vi "Camera Parameter to 3D Projection Matrix.vi"(0 "Size":T2, 1 "Far (Default: 100)":dbl=100.0 format="%#_13g", 3 "Camera Matrix":T1, 4 "Near (Default: 0.01)":dbl=0.01 format="%#_13g") -> (2 "Bounds":T3, 5 "3D-Control Projection Matrix":sgl[][](array[numeric]))   [LabVIEW 2020, in "g_ar_toolkit.ar.lvlib"]
uses:
  g_ar_toolkit.ar.lvlib
  <vilib>/Utility/miscctls.llb/LVBoundsTypeDef.ctl
  g_ar_toolkit.common/Image Size (Integer).ctl
  g_ar_toolkit.common/Camera Matrix.ctl
  g_ar_toolkit.common/g_ar_toolkit.common.lvlib
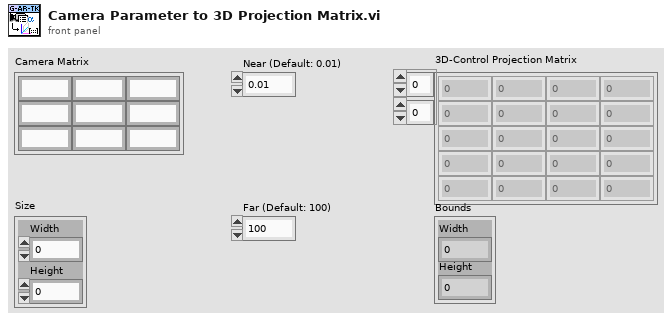
[diagram p1: front panel]
types:
  T1 = typedef "g_ar_toolkit.common.lvlib/Camera Matrix.ctl" = cluster{"m 0,0":dbl, "m 0,1":dbl, "m 0,2":dbl, "m 1,0":dbl, "m 1,1":dbl, "m 1,2":dbl, "m 2,0":dbl, "m 2,1":dbl, "m 2,2":dbl}
  T2 = typedef "g_ar_toolkit.common.lvlib/Image Size (Integer).ctl" = cluster{"Width":u16, "Height":u16}
  T3 = typedef "LVBoundsTypeDef.ctl" = cluster{"Width":u32, "Height":u32}
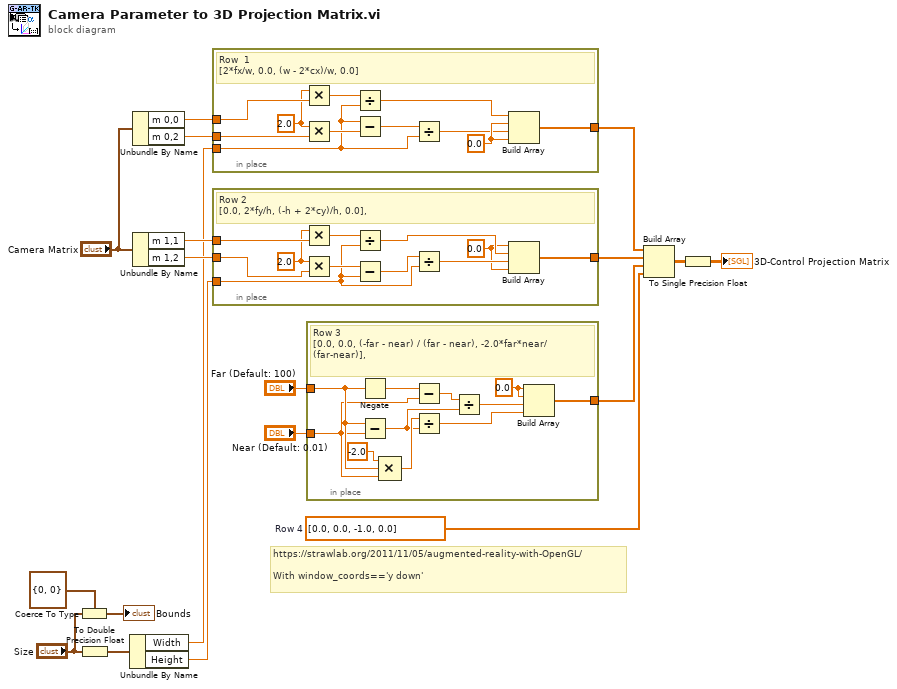
[diagram p0: block diagram]
diagram:
  w17 = dbl[] [0.0, 0.0, -1.0, 0.0]  # Row 4
  # "https://strawlab.org/2011/11/05/augmented-reality-with-OpenGL/\n\nWith window_coords=='y down'"
  n1 = Coerce To Type(0:"Size", 1:T3 {"Width"=0, "Height"=0} ("Content Bounds")) -> (2:→"Bounds":T3)
  n2 = To Double Precision Float(number="Size") -> (double precision float=w3:cluster{"Width":dbl, "Height":dbl})
  n3 = Unbundle By Name(w3) -> ("Width"=w5:dbl, "Height"=w4:dbl)
  n4 = Unbundle By Name("Camera Matrix") -> ("m 0,0"=w15:dbl, "m 0,2"=w14:dbl)
  n5 = Unbundle By Name("Camera Matrix") -> ("m 1,1"=w13:dbl, "m 1,2"=w12:dbl)
  n6 = in-place {
    in-place-border: [w29] -> w16
    in-place-border: w15 -> [w28]
    in-place-border: w14 -> [w22]
    in-place-border: w5 -> [w20]
    w23 = 2.0
    w30 = 0.0 ("element")
    # "Row  1\n[2*fx/w, 0.0, (w - 2*cx)/w, 0.0]"
    n7 = Multiply(x=w23, y=w28) -> (x*y=w26:dbl)
    n8 = Multiply(x=w23, y=w22) -> (x*y=w21:dbl)
    n9 = Divide(x=w26, y=w20) -> (x/y=w27:dbl)
    n10 = Subtract(x=w20, y=w21) -> (x-y=w25:dbl)
    n11 = Divide(x=w25, y=w20) -> (x/y=w24:dbl)
    n12 = Build Array(w27, w30, w24, w30) -> (w29:dbl[])
  }
  n13 = in-place {
    in-place-border: [w41] -> w11
    in-place-border: w13 -> [w39]
    in-place-border: w4 -> [w34]
    in-place-border: w12 -> [w37]
    w38 = 2.0
    w32 = 0.0 ("element")
    # "Row 2\n[0.0, 2*fy/h, (-h + 2*cy)/h, 0.0],"
    n14 = Multiply(x=w38, y=w39) -> (x*y=w40:dbl)
    n15 = Multiply(x=w38, y=w37) -> (x*y=w35:dbl)
    n16 = Divide(x=w40, y=w34) -> (x/y=w36:dbl)
    n17 = Subtract(x=w35, y=w34) -> (x-y=w31:dbl)
    n18 = Divide(x=w31, y=w34) -> (x/y=w33:dbl)
    n19 = Build Array(w32, w36, w33, w32) -> (w41:dbl[])
  }
  n20 = in-place {
    in-place-border: [w52] -> w10
    in-place-border: "Far (Default: 100)" -> [w47]
    in-place-border: "Near (Default: 0.01)" -> [w46]
    w51 = 0.0 ("element")
    # "Row 3\n[0.0, 0.0, (-far - near) / (far - near), -2.0*far*near/(far-near)],"
    n21 = Negate(x=w47) -> (-x=w50:dbl)
    n22 = Subtract(x=w47, y=w46) -> (x-y=w43:dbl)
    n23 = Compound Arithmetic op=MULTIPLY(-2.0 ("x"), w47, w46) -> (w44:dbl)
    n24 = Subtract(x=w50, y=w46) -> (x-y=w49:dbl)
    n25 = Divide(x=w44, y=w43) -> (x/y=w42:dbl)
    n26 = Divide(x=w49, y=w43) -> (x/y=w48:dbl)
    n27 = Build Array(w51, w51, w48, w42) -> (w52:dbl[])
  }
  n28 = Build Array(w16, w11, w10, w17) -> (w7:dbl[][])
  n29 = To Single Precision Float(number=w7) -> (single precision float=→"3D-Control Projection Matrix":sgl[][])
